vi "Plot Example.vi"() -> ()   [LabVIEW 2015, in "VC940.lvlib"]
uses:
  VC940.lvlib
panel:
  in  "Clear":bool
  out "XY Graph":cluster{dbl[], dbl[]}(graph)
  out "Connection":bool
  out "Display":string
  in  "Port name":string="COM1"
  in  "Exit":bool
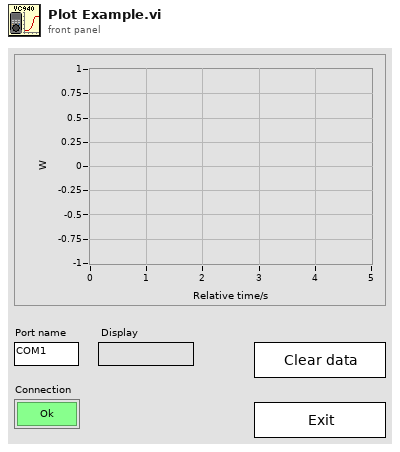
[diagram p1: front panel]
types:
  T1 = typedef "VC940.lvlib/Function.ctl" = enum8{"mV AC", "V DC", "V AC", "mV DC", "Ohm", "nF", "°C", "µA", "mA", "A", "Ohm Fm", "V Diode", "Hz", "°F", "W", "%4-20mA"}
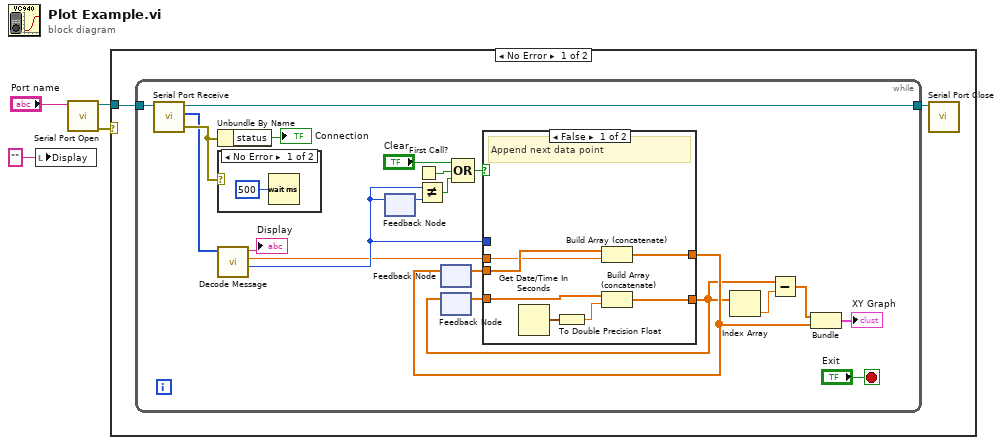
[diagram p0: block diagram]
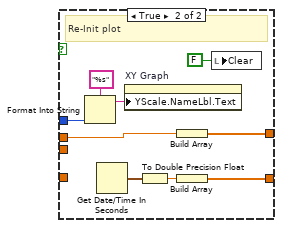
[diagram p2: hidden frame]
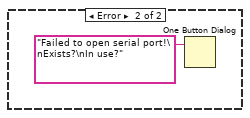
[diagram p4: hidden frame]
diagram:
  n1 = local write "Display"("" ("Data")) -> ()
  n2 = call "Serial Port Open.vi"("Port name (COM1)"="Port name") -> ("error out"=w1:errorcluster, "Port handle"=w3:refnum<k24>)  [unwired: 9 in]
  n3 = case shown="No Error" w1 {
    tunnel: w3 -> [w6 _]
    frame No Error {
      n4 = while {
        tunnel: w6 -> [w26]
        tunnel: [w25] -> w5
        stop <- "Exit" stop-if-true
        n5 = call "Serial Port Receive.vi"("Port handle in"=w26) -> ("error out"=w23:errorcluster, "Message"=w21:u8[], "Port handle out"=w25:refnum<k24>)  [unwired: 8 in]
        n6 = Unbundle By Name(w23) -> ("status"=→"Connection":bool)
        n7 = case shown="No Error" w23 {
          frame No Error {
            n8 = Wait (ms)(milliseconds to wait=u32 500) -> ()  [unwired: 1 out]
          }
          frame Error {
          }
        }
        n9 = call "Decode Message.vi"("Message"=w21) -> ("Function (0..15)"=w16:T1, "Value"=w14:dbl, "Display string"=→"Display":string)  [unwired: 5 in, 3 out]
        n10 = feedback-in #1(w16) -> ()
        n11 = feedback #1() -> (w20:T1)  [unwired: 1 in]
        n12 = First Call?() -> (First Call?: T/F=w19:bool)
        n13 = Not Equal?(x=w16, y=w20) -> (x != y?=w18:bool)
        n14 = feedback #2() -> (w13:dbl[])  [unwired: 1 in]
        n15 = feedback #3() -> (w15:dbl[])  [unwired: 1 in]
        n16 = Compound Arithmetic op=OR("Clear", w19, w18) -> (w17:bool)
        n17 = case shown="False" w17 {
          tunnel: w16 -> [_ w43]
          tunnel: w15 -> [w34 _]
          tunnel: [w33 w39] -> w9
          tunnel: w14 -> [w31 w38]
          tunnel: [w30 w37] -> w12
          tunnel: w13 -> [w32 _]
          frame False {
            # "Append next data point"
            n18 = Get Date/Time In Seconds() -> (seconds since 1Jan1904=w29:timestamp)
            n19 = To Double Precision Float(number=w29) -> (double precision float=w28:dbl)
            n20 = Build Array (concatenate)(w32, w31) -> (w30:dbl[])
            n21 = Build Array (concatenate)(w34, w28) -> (w33:dbl[])
          }
          frame True {
            # "Re-Init plot"
            n22 = Format Into String(format string="%s", w43) -> (resulting string=w41:string)  [unwired: 2 in, 1 out]
            n23 = Get Date/Time In Seconds() -> (seconds since 1Jan1904=w40:timestamp)
            n24 = property on="XY Graph" class="XYGraph (strict)"("YScale.NameLbl.Text"=w41) -> ()  [unwired: 2 in, 2 out]
            n25 = To Double Precision Float(number=w40) -> (double precision float=w36:dbl)
            n26 = Build Array(w38) -> (w37:dbl[])
            n27 = Build Array(w36) -> (w39:dbl[])
            n28 = local write "Clear"(FALSE ("Clear")) -> ()
          }
        }
        n29 = feedback-in #2(w12) -> ()
        n30 = feedback-in #3(w9) -> ()
        n31 = Index Array(array=w9) -> (element=w10:dbl)  [unwired: 1 in]
        n32 = Subtract(x=w9, y=w10) -> (x-y=w8:dbl[])
        n33 = Bundle(w8, w12) -> (→"XY Graph":cluster{dbl[], dbl[]})  [unwired: 1 in]
      }
      n34 = call "Serial Port Close.vi"("Port handle"=w5) -> ()  [unwired: 10 in, 1 out]
    }
    frame Error {
      n35 = One Button Dialog(message="Failed to open serial port!\nExists?\nIn use?") -> ()  [unwired: 1 in, 1 out]
    }
  }
